vi "subviprogram.vi"() -> (2 "Array 2":i32[](array[numeric]), 3 "Numeric 2":i32)   [LabVIEW 2019]
uses:
  subglobalbooleanmanueel.vi
  <vilib>/myRIO/Common/Instrument Driver Framework/myRIO v1.0/DIO/typedefs/DIO Channels Enum.ctl
  <vilib>/myRIO/Common/Instrument Driver Framework/myRIO v1.0/DIO/typedefs/DIO Channels List.ctl
  <vilib>/myRIO/Common/Instrument Driver Framework/Utilities/typedefs/Generic FPGA Reference.ctl
  <vilib>/myRIO/Common/Instrument Driver Framework/Utilities/typedefs/myRIO v1.0 Reference.ctl
  <vilib>/myRIO/Common/Instrument Driver Framework/Utilities/typedefs/Hardware Version Enum.ctl
  <vilib>/myRIO/Common/Instrument Driver Framework/Utilities/typedefs/myRIO Generic Hardware Reference.ctl
  <vilib>/myRIO/Instrument Drivers/Onboard IO/DIO/typedefs/DIO Reference.ctl
  <vilib>/myRIO/Instrument Drivers/Onboard IO/DIO/DIO.lvlib
  <vilib>/myRIO/Instrument Drivers/Onboard IO/DIO/vis/Read.vi
  <vilib>/userDefined/High Color/nirio_resource_hc.ctl
  <vilib>/myRIO/Common/Instrument Driver Framework/myRIO v1.0/DIO/vis/myRIO v1.1 Open DIO.vi
  <vilib>/myRIO/Instrument Drivers/Onboard IO/DIO/vis/myRIO DIO Open.xnode
  <vilib>/myRIO/Common/Instrument Driver Framework/Utilities/vis/Is FPGA Ref Available.vi
  <vilib>/myRIO/Express VI/Onboard IO/DI/DI Express VI.xnode
  <vilib>/myRIO/Common/Instrument Driver Framework/Utilities/typedefs/Analog Scaling Constants.ctl
  <vilib>/myRIO/Common/Instrument Driver Framework/Utilities/typedefs/Analog Scaling Constants List.ctl
  <vilib>/myRIO/Common/Instrument Driver Framework/myRIO v1.0/AO/typedefs/AO Channels Enum.ctl
  <vilib>/myRIO/Common/Instrument Driver Framework/myRIO v1.0/AO/typedefs/AO Channels List.ctl
  <vilib>/myRIO/Instrument Drivers/Onboard IO/AO/typedefs/AO Reference.ctl
  <vilib>/myRIO/Instrument Drivers/Onboard IO/AO/AO.lvlib
  <vilib>/myRIO/Instrument Drivers/Onboard IO/AO/vis/Write.vi
  <vilib>/myRIO/Common/Instrument Driver Framework/myRIO v1.0/AO/vis/myRIO v1.1 Open AO.vi
  <vilib>/myRIO/Instrument Drivers/Onboard IO/AO/vis/myRIO AO Open.xnode
  <vilib>/myRIO/Express VI/Onboard IO/AO/AO Express VI.xnode
panel:
  out "Boolean manueel":bool
  in  "STOP":bool
  in  "tijdsinterval 8":dbl
  in  "tijdsinterval 7":dbl
  in  "tijdsinterval 6":dbl
  in  "tijdsinterval 5":dbl
  in  "tijdsinterval 4":dbl
  in  "tijdsinterval 3":dbl
  in  "tijdsinterval 2":dbl
  out "groen":u32
  out "rood":u32
  out "error out 3":errorcluster
  in  "error in (no error) 3":errorcluster
  in  "stoppen":bool
  in  "rechts draaien achteruit":bool
  in  "links draaien achteruit":bool
  out "appended array":dbl[](array[numeric])
  in  "snelheid":dbl
  in  "rechts draaien":bool
  in  "links draaien":bool
  in  "achterwaarts":bool
  in  "voorwaarts":bool
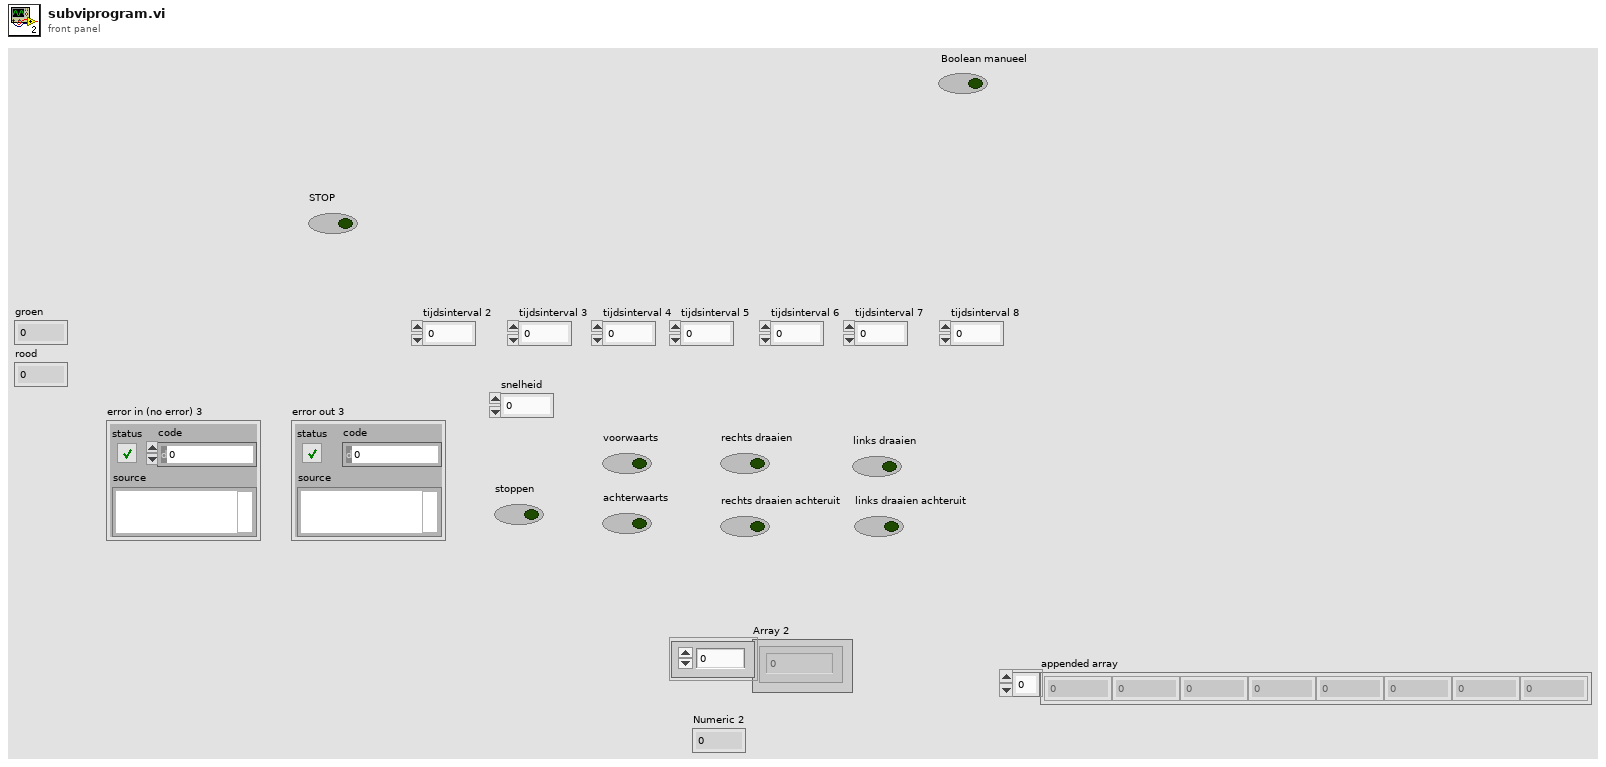
[diagram p1: front panel]
types:
  T1 = typedef "DIO.lvlib/DIO Reference.ctl" = cluster{"myRIO Reference":T2, "DIO Channels List":T6}
  T2 = typedef "myRIO Generic Hardware Reference.ctl" = cluster{"myRIO Model":T3, "myRIO Hardware Reference":T4}
  T3 = typedef "Hardware Version Enum.ctl" = enum16{"Unknown", "myRIO-1900", "myRIO-1950", "roboRIO", "NI ELVIS RIO CM", "ELVIS III"}
  T4 = typedef "myRIO v1.0 Reference.ctl" = cluster{"Generic FPGA Reference":T5, "Allow multiple opens":bool}
  T5 = typedef "Generic FPGA Reference.ctl" = refnum<k20>
  T6 = typedef "DIO Channels List.ctl" = T7[]
  T7 = typedef "DIO Channels Enum.ctl" = enum16{"Not Connected", "C/DIO0", "C/DIO1", "C/DIO2", "C/DIO3", "C/DIO4", "C/DIO5", "C/DIO6", "C/DIO7", "A/DIO0", "A/DIO1", "A/DIO2", "A/DIO3", "A/DIO4", "A/DIO5", "A/DIO6", "A/DIO7", "A/DIO8", "A/DIO9", "A/DIO10", "A/DIO11", "A/DIO12", "A/DIO13", "A/DIO14", "A/DIO15", "A/DIO16", "A/DIO17", "A/DIO18", "A/DIO19", "B/DIO0", "B/DIO1", "B/DIO2", "B/DIO3", "B/DIO4", "B/DIO5", "B/DIO6", "B/DIO7", "B/DIO8", "B/DIO9", "B/DIO10", "B/DIO11", "B/DIO12", "B/DIO13", "B/DIO14", "B/DIO15", "B/DIO16", "B/DIO17", "B/DIO18", "B/DIO19", "LED0", "LED1", "LED2", "LED3", "Button0", "DIO/DIO0", "DIO/DIO1", "DIO/DIO2", "DIO/DIO3", "DIO/DIO4", "DIO/DIO5", "DIO/DIO6", "DIO/DIO7", "DIO/DIO8", "DIO/DIO9", "SPI/CS0", "SPI/CS1", "SPI/CS2", "SPI/CS3", "LED RADIO (Green)", "LED RADIO (Red)", "LED COMM (Green)", "LED COMM (Red)", "LED MODE (Green)", "LED MODE (Red)"}
  T8 = typedef "nirio_resource_hc.ctl" = tag
  T9 = typedef "AO.lvlib/AO Reference.ctl" = cluster{"myRIO Reference":T2, "AO Channel List":T10, "AO Scaling Constant List":T12}
  T10 = typedef "AO Channels List.ctl" = T11[]
  T11 = typedef "AO Channels Enum.ctl" = enum16{"Not Connected", "AudioOut/Left", "AudioOut/Right", "C/AO0", "C/AO1", "A/AO0", "A/AO1", "B/AO0", "B/AO1"}
  T12 = typedef "Analog Scaling Constants List.ctl" = T13[]
  T13 = typedef "Analog Scaling Constants.ctl" = cluster{"LSB Weight (Volts)":dbl, "Offset (Volts)":dbl, "Signed?":bool}
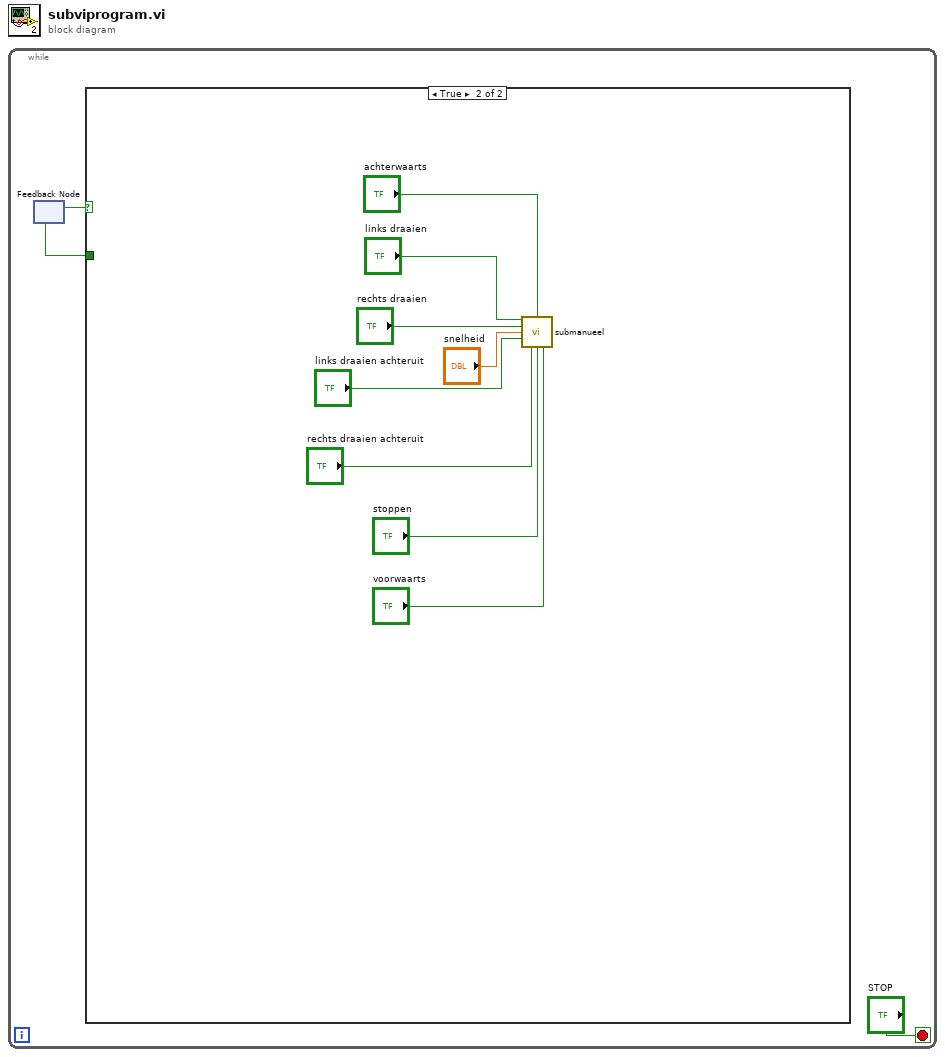
[diagram p0: block diagram]
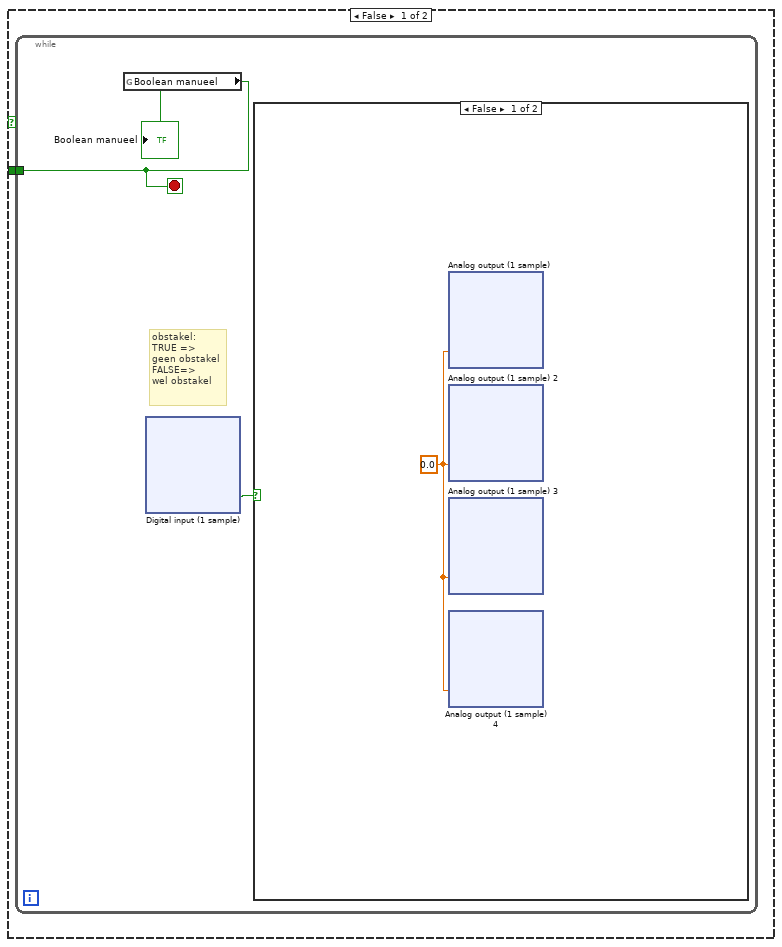
[diagram p2: hidden frame]
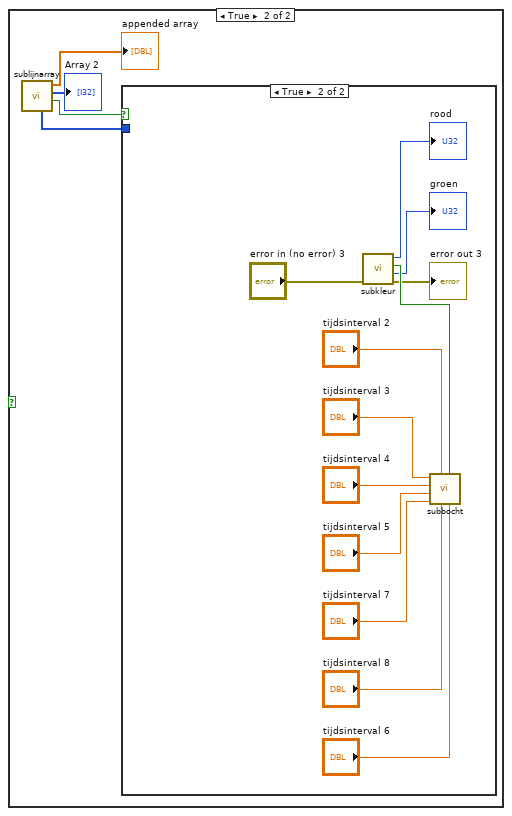
[diagram p3: hidden frame]
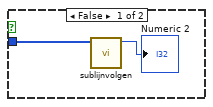
[diagram p4: hidden frame]
diagram:
  n1 = while {
    stop <- "STOP" stop-if-true
    n2 = feedback #1() -> (w1:bool)  [unwired: 1 in]
    n3 = case shown="True" w1 {
      tunnel: [w4 _] -> w2
      frame False {
        n4 = while {
          tunnel: [w6] -> w4
          stop <- w6 stop-if-true
          # "obstakel:\nTRUE => \ngeen obstakel\nFALSE=>\nwel obstakel"
          n5 = global read "subglobalbooleanmanueel.vi" "Boolean manueel"() -> (w6:bool)
          "Boolean manueel" <- w6
          n6 = xnode "Digital input (1 sample)"() -> ("A/DIO1 (Pin 13)"=w5:bool)  [unwired: 1 in, 1 out]
          n7 = case shown="False" w5 {
            frame False {
              w42 = 0.0
              n8 = xnode "Analog output (1 sample)"("A/AO0 (Pin 2)"=w42) -> ()  [unwired: 1 in, 1 out]
              n9 = xnode "Analog output (1 sample) 2"("A/AO1 (Pin 4)"=w42) -> ()  [unwired: 1 in, 1 out]
              n10 = xnode "Analog output (1 sample) 3"("B/AO0 (Pin 2)"=w42) -> ()  [unwired: 1 in, 1 out]
              n11 = xnode "Analog output (1 sample) 4"("B/AO1 (Pin 4)"=w42) -> ()  [unwired: 1 in, 1 out]
            }
            frame True {
              n12 = call "sublijnarray.vi"() -> ("Boolean"=w193:bool, "Array 2"=→"Array 2":i32[], "appended array"=→"appended array":dbl[], "Array"=w194:i32[])  [unwired: 8 in]
              n13 = case shown="True" w193 {
                tunnel: w194 -> [w196 _]
                frame False {
                  n14 = call "sublijnvolgen.vi"("Array"=w196) -> ("Numeric 2"=→"Numeric 2":i32)  [unwired: 10 in]
                }
                frame True {
                  n15 = call "subkleur.vi"("error in (no error)"="error in (no error) 3") -> ("error out"=→"error out 3":errorcluster, "groen"=→"groen":u32, "Boolean"=w208:bool, "rood"=→"rood":u32)  [unwired: 7 in]
                  n16 = call "subbocht.vi"("tijdsinterval 6"="tijdsinterval 6", "Boolean"=w208, "tijdsinterval 8"="tijdsinterval 8", "tijdsinterval in"="tijdsinterval 2", "tijdsinterval 7"="tijdsinterval 7", "tijdsinterval 5"="tijdsinterval 5", "tijdsinterval 4"="tijdsinterval 4", "tijdsinterval 3"="tijdsinterval 3") -> ()  [unwired: 4 in]
                }
              }
            }
          }
        }
      }
      frame True {
        n17 = call "submanueel.vi"("links draaien"="links draaien", "achterwaarts"="achterwaarts", "rechts draaien"="rechts draaien", "snelheid"="snelheid", "links draaien achteruit"="links draaien achteruit", "rechts draaien achteruit"="rechts draaien achteruit", "stoppen"="stoppen", "voorwaarts"="voorwaarts") -> ()  [unwired: 8 in]
      }
    }
    n18 = feedback-in #1(w2) -> ()
  }
